vi "Micronix Approach Main.vi"() -> ()   [LabVIEW 2021]
panel:
  in  "Polarity":bool caption="pos      neg"
  in  "Controller #":string
  in  "Pulse In":tag
  in  "rate":dbl=1000.0
  in  "Reset":bool
  in  "Stop":bool
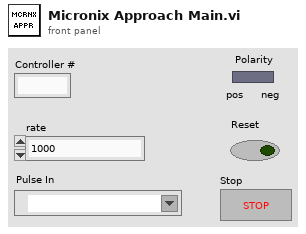
[diagram p1: front panel]
types:
  T1 = cluster{"P type":u16, "VISA resource name out":refnum<visa-resource-name>, " Terminator":string, "Timeout":i32}
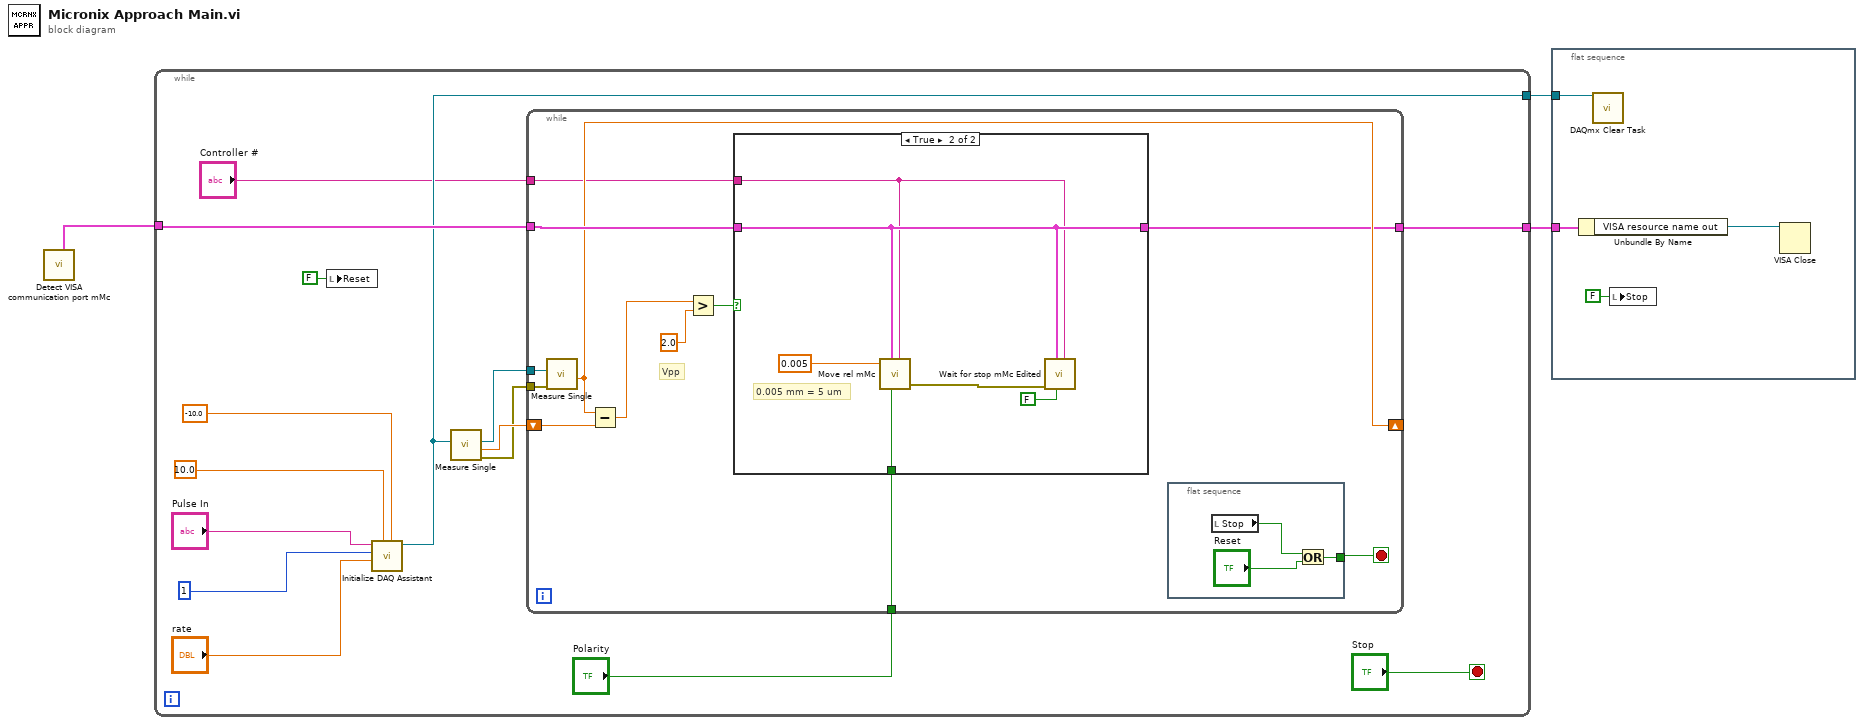
[diagram p0: block diagram]
diagram:
  n1 = call "Detect VISA communication port mMc.vi"() -> ("Port"=w3:T1)  [unwired: 6 in, 3 out]
  n2 = while {
    tunnel: w3 -> [w17]
    tunnel: [w9] -> w2
    tunnel: [w10] -> w1
    stop <- "Stop" stop-if-true
    n3 = local write "Reset"(FALSE ("Reset")) -> ()
    n4 = call "Initialize DAQ Assistant.vi"("minimum value"=-10.0, "maximum value"=10.0, "rate"="rate", "number of samples"=1, "physical channels"="Pulse In") -> ("task out"=w9:refnum<k21>)  [unwired: 5 in, 1 out]
    n5 = call "Measure Single.vi"("task/channels in"=w9) -> ("error out"=w13:errorcluster, "Value"=w14:dbl, "task out"=w4:refnum<k21>)  [unwired: 8 in]
    n6 = while {
      tunnel: w17 -> [w30]
      shift-right: [w24] -> _
      shift-left: w14 -> [w29]
      tunnel: w4 -> [w26]
      tunnel: w13 -> [w25]
      tunnel: [w22] -> w10
      tunnel: "Controller #" -> [w21]
      tunnel: "Polarity" -> [w20]
      stop <- w23 stop-if-true
      # "Vpp"
      n7 = call "Measure Single.vi"("error in"=w25, "task/channels in"=w26) -> ("Value"=w24:dbl)  [unwired: 7 in, 2 out]
      n8 = Subtract(x=w24, y=w29) -> (x-y=w19:dbl)
      n9 = Greater?(x=w19, y=2.0) -> (0:w28:bool)
      n10 = case shown="True" w28 {
        tunnel: w30 -> [w34 w37]
        tunnel: [w34 w37] -> w22
        tunnel: w21 -> [_ w35]
        tunnel: w20 -> [_ w36]
        frame False {
        }
        frame True {
          # "0.005 mm = 5 um"
          n11 = call "Move rel mMc.vi"("position incr"=0.005, "Port"=w37, "rev dir?"=w36, "Controller #"=w35) -> ("error out"=w40:errorcluster)  [unwired: 5 in]
          n12 = call "Wait for stop mMc Edited.vi"("Controller #"=w35, "wait for in pos"=FALSE, "Port"=w37, "error in (no error)"=w40) -> ()  [unwired: 7 in, 1 out]
        }
      }
      n13 = flat-sequence {
        tunnel: [w33] -> w23
        frame #0 {
          n14 = local read "Stop"() -> (w31:bool)
          n15 = Or(x=w31, y="Reset") -> (x .or. y?=w33:bool)
        }
      }
    }
  }
  n16 = flat-sequence {
    tunnel: w2 -> [w44]
    tunnel: w1 -> [w42]
    frame #0 {
      n17 = Unbundle By Name(w42) -> ("VISA resource name out"=w43:refnum<visa-resource-name>)
      n18 = call <vilib>:"DAQmx Clear Task.vi"("task in"=w44) -> ()  [unwired: 14 in, 1 out]
      n19 = local write "Stop"(FALSE ("Stop")) -> ()
      n20 = VISA Close(VISA resource name=w43) -> ()  [unwired: 1 in, 1 out]
    }
  }
